vi "CPP_ContineAfterDisplayPosAndWait.vi"() -> (5 "Plug in titles":string[](array[string]), 7 "Plug in values":string[](array[string]))   [LabVIEW 2011]
uses:
  Controls/Analysis_info_cluster.ctl
  Controls/Inst_type.ctl
  Controls/Instrument_Array.ctl
  Globals/Plug_in_data_global.vi
  Globals/Meas_global.vi
  Globals/ForceWait.vi
panel:
  in  "ForceWait":bool
  out "Analysis Info cluster":T1[](array[typedef])=[{"Colour"=0, "Inst type"=enum."Pitot-static tube", "Inst name"="Manometer voltage", "Symbol"="U", "Code name"="", "Extra Info"="U", "Inst Array"=enum."PWA", "Index"=0, "Voltage Index"=0, "Extra Titles"=[], "Extra Values"=[]}, {"Colour"=0, "Inst type"=enum."Pitot-static tube", "Inst name"="Manometer voltage", "Symbol"="U", "Code name"="", "Extra Info"="U", "Inst Array"=enum."PWA", "Index"=0, "Voltage Index"=0, "Extra Titles"=[], "Extra Values"=[]}, {"Colour"=0, "Inst type"=enum."Pitot-static tube", "Inst name"="Manometer voltage", "Symbol"="U", "Code name"="", "Extra Info"="U", "Inst Array"=enum."PWA", "Index"=0, "Voltage Index"=0, "Extra Titles"=[], "Extra Values"=[]}, {"Colour"=0, "Inst type"=enum."Pitot-static tube", "Inst name"="Manometer voltage", "Symbol"="U", "Code name"="", "Extra Info"="U", "Inst Array"=enum."PWA", "Index"=0, "Voltage Index"=0, "Extra Titles"=[], "Extra Values"=[]}]
  out "Current Block No":i32
  out "Raw data file":path
  out "Actual Sampling rate (Hz)":dbl=1000.0 format="%.2f"
  out "Equi Spaced":dbl[][](array[numeric]) format="%.2f"
  # "You must have just these two indicators on the connector pane of the vi"
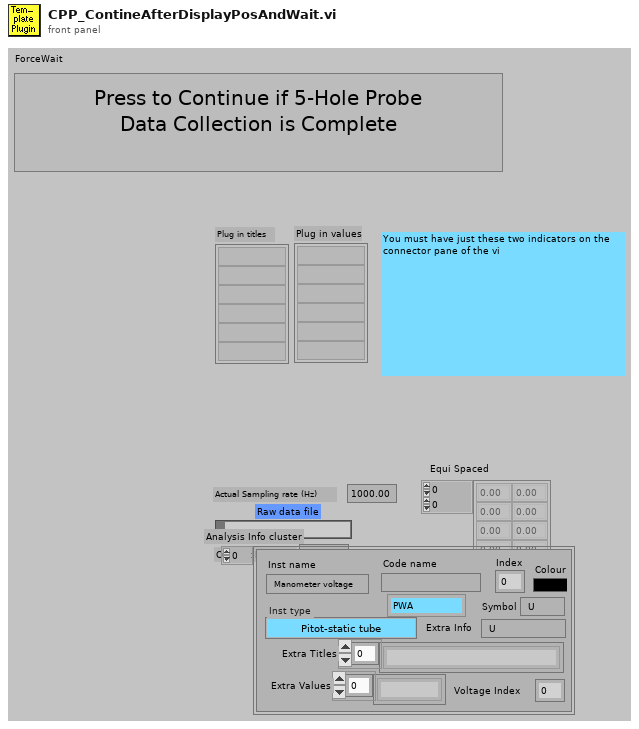
[diagram p1: front panel]
types:
  T1 = typedef "Analysis_info_cluster.ctl" = cluster{"Colour":u32, "Inst type":T2, "Inst name":string, "Symbol":string, "Code name":string, "Extra Info":string, "Inst Array":T3, "Index":i32, "Voltage Index":i32, "Extra Titles":string[], "Extra Values":string[]}
  T2 = typedef "Inst_type.ctl" = enum16{"Propeller anemometer", "Raw voltage", "Pressure Transducer", "Pitot-static tube", "Preston tube", "Hot wire", "Cross wire 1", "Cross wire 2", "Generic Linear", "Generic Polynomial", "Generic BackPoly", "Fast FID", "Thermocouple", "Cold wire", "Pulsed Wire", "LDA Vel", "LDA Tran time", "LDA Arr time"}
  T3 = typedef "Instrument_Array.ctl" = enum16{"PWA", "LDA", "Analogue"}
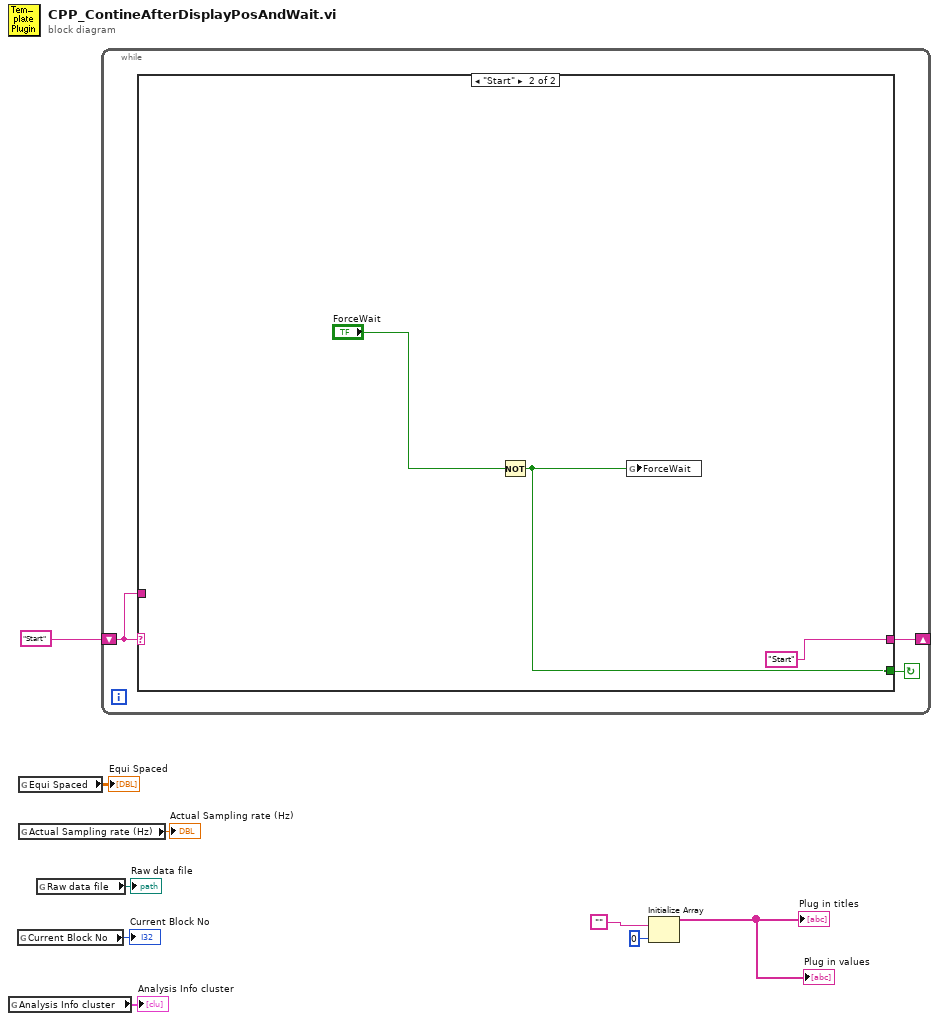
[diagram p0: block diagram]
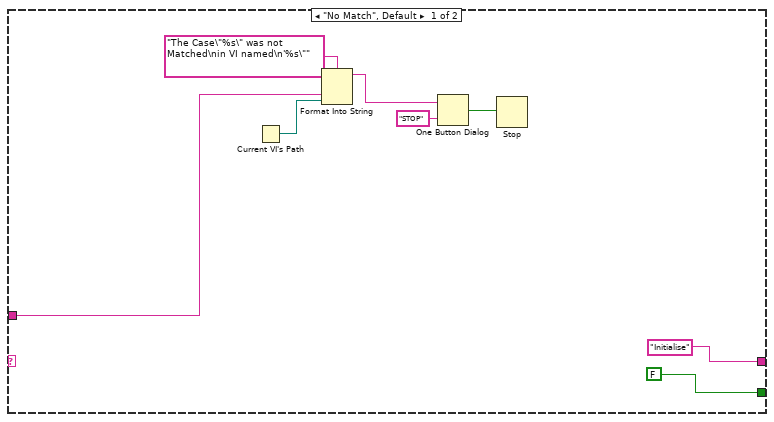
[diagram p2: hidden frame]
diagram:
  n1 = global read "Meas_global.vi" "Analysis Info cluster"() -> (→"Analysis Info cluster":T1[])
  n2 = global read "Meas_global.vi" "Current Block No"() -> (→"Current Block No":i32)
  n3 = global read "Plug_in_data_global.vi" "Equi Spaced"() -> (→"Equi Spaced":dbl[][])
  n4 = global read "Meas_global.vi" "Actual Sampling rate (Hz)"() -> (→"Actual Sampling rate (Hz)":dbl)
  n5 = global read "Meas_global.vi" "Raw data file"() -> (→"Raw data file":path)
  n6 = while {
    shift-left: "Start" -> [w10]
    shift-right: [w11] -> _
    stop <- w12 continue-if-true
    n7 = case shown="\"Start\"" w10 {
      tunnel: [FALSE w21] -> w12
      tunnel: ["Initialise" "Start"] -> w11
      tunnel: w10 -> [w15 _]
      frame "No Match", Default {
        n8 = Current VI's Path() -> (path=w14:path)
        n9 = Format Into String(format string="The Case\"%s\" was not Matched\nin VI named\n'%s\"" ("Format String"), w15, w14) -> (resulting string=w18:string)  [unwired: 2 in, 1 out]
        n10 = One Button Dialog(message=w18, button name ("OK")="STOP") -> (true=w16:bool)
        n11 = Stop(stop? (T)=w16) -> ()
      }
      frame "Start" {
        n12 = Not(x="ForceWait") -> (.not. x?=w21:bool)
        n13 = global write "ForceWait.vi" "ForceWait"(w21) -> ()
      }
    }
  }
  n14 = Initialize Array("", 0) -> (→"Plug in values" →"Plug in titles":string[])
